vi "SVA_MAIN_2.vi"() -> ()   [LabVIEW 2021]
uses:
  Control-Case.ctl
  <vilib>/vision/NI_Vision_Development_Module.lvlib
panel:
  out "Distance 2":dbl[](graph) caption="Distancia entre perfil ideal y perfil real"
  out "Distance":dbl[](graph) caption="Distancia entre perfil ideal y perfil real"
  out "new picture 2":picture
  out "new picture":picture
  out "Datos finales":T1(array[cluster])
  in  "Crear patrón":bool
  in  "Concluir":bool
  in  "Lateral":bool
  in  "Superior":bool
  out "Fecha final":timestamp
  out "Rechazadas":dbl
  out "Aprobadas":dbl
  in  "Valor de aprobación Superiror":dbl=4.0 min=0.0 format="%.2f"
  out "Fecha inicio":timestamp
  out "Muestras":i16
  in  "Valor de aprobación Frontal":dbl=4.0 min=0.0 format="%.2f"
  # "Descripción:\nEste instrumento virtual permite detectar irregularidades en la geometría de latas de refresco usando el análisis de contornos:\n-Primeramente debe obtenerse un patrón para el perfil lateral e caso de no tenerlo, pues este se usará para detectar las irregularidades de capturas posteriores.\n-Como siguiente paso se toma una captura del perfil lateral y esta se desplegará en la imagen izquierda.\n-Como siguiente paso se toma una captura del perfil superior y esta se desplegará en la imagen derecha."
  # "Sistema de detección de defectos en latas \nbasado en el análisis de contornos\nProyecto de fin de semestre \nSistemas de visión artificial\nProfesor Erick Huitrón Ramírez"
  # "CUEVAS CERÓN SERGIO ALBERTO\nREYES PÉREZ JAVIER\nSALCEDO LICEA JUAN CARLOS"
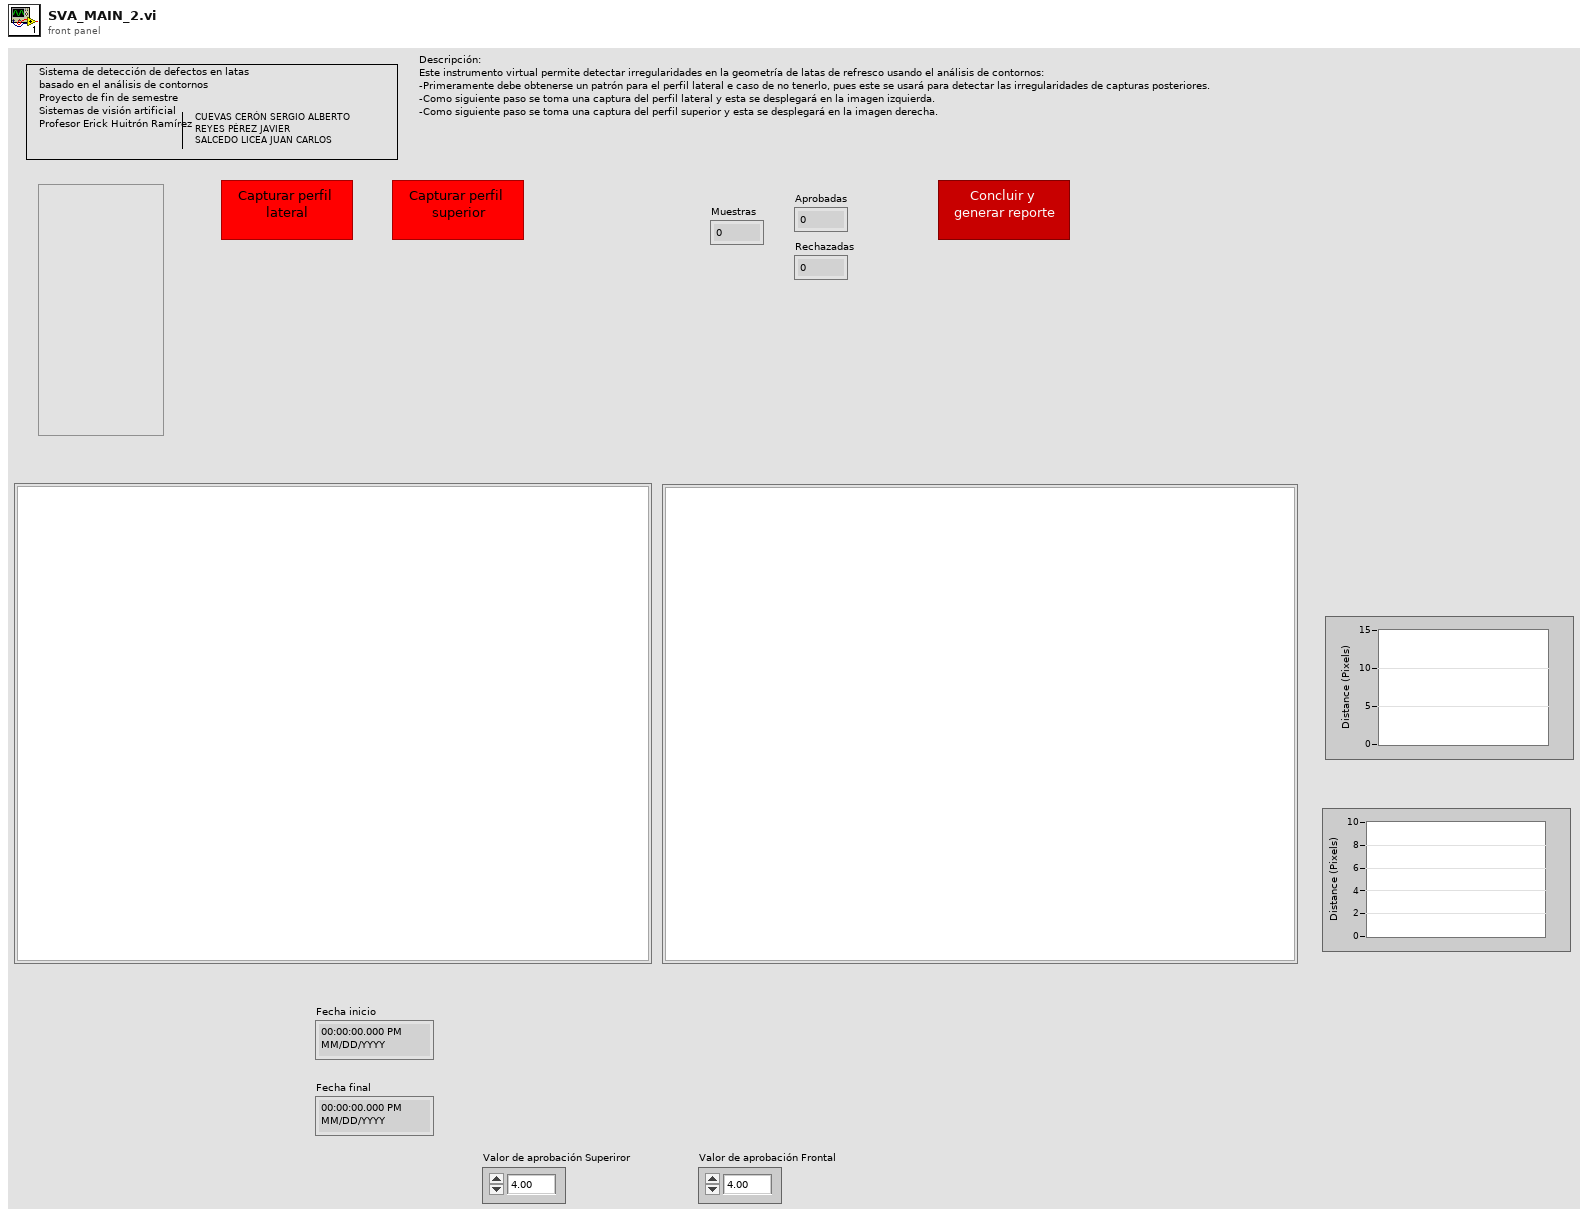
[diagram p1: front panel]
types:
  T1 = cluster{"Class":string, string, string, string}[]
  T2 = typedef "Control-Case.ctl" = enum16{"Espera", "Patrón", "Toma lateral", "Toma superior", "Concluir"}
  T3 = enum16{"Rect Left To Right", "Rect Right To Left", "Rect Top To Bottom", "Rect Bottom To Top", "Annulus Inner To Outer", "Annulus Outer To Inner", "Annulus Start Angle To End Angle", "Annulus End Angle To Start Angle"}
  T4 = enum16{"Closest To Search Start", "Maximum Length", "Strongest Mean Gradient Change"}
  T5 = cluster{"Overlay?":bool, "Color":u32, "Width":u32, "Maintain Width?":bool}
  T6 = typedef "IMAQ Rectangle" = cluster{"Left":i32, "Top":i32, "Right":i32, "Bottom":i32, "Rotation":dbl}
  T7 = typedef "IMAQ Image.ctl" = refnum<image>
  T8 = typedef "ROI Descriptor" = cluster{"Global Rectangle":i32[], "Contours":cluster{"ID":enum32{"External", "Internal"}, "Type":u32, "Coordinates":i32[]}[]}
  T9 = cluster{"Distance (Pixels)":dbl, "Distance (Real World)":dbl, "Angle (Absolute)":dbl, "Angle (Relative)":dbl}
  T10 = cluster{"Target Point":cluster{"X":dbl, "Y":dbl}, "Template Point":cluster{"X":dbl, "Y":dbl}, "Distance":dbl}[]
  T11 = cluster{"Class":string, "Distance (Pixels)":dbl, bool, "Distance (Pixels)":dbl}
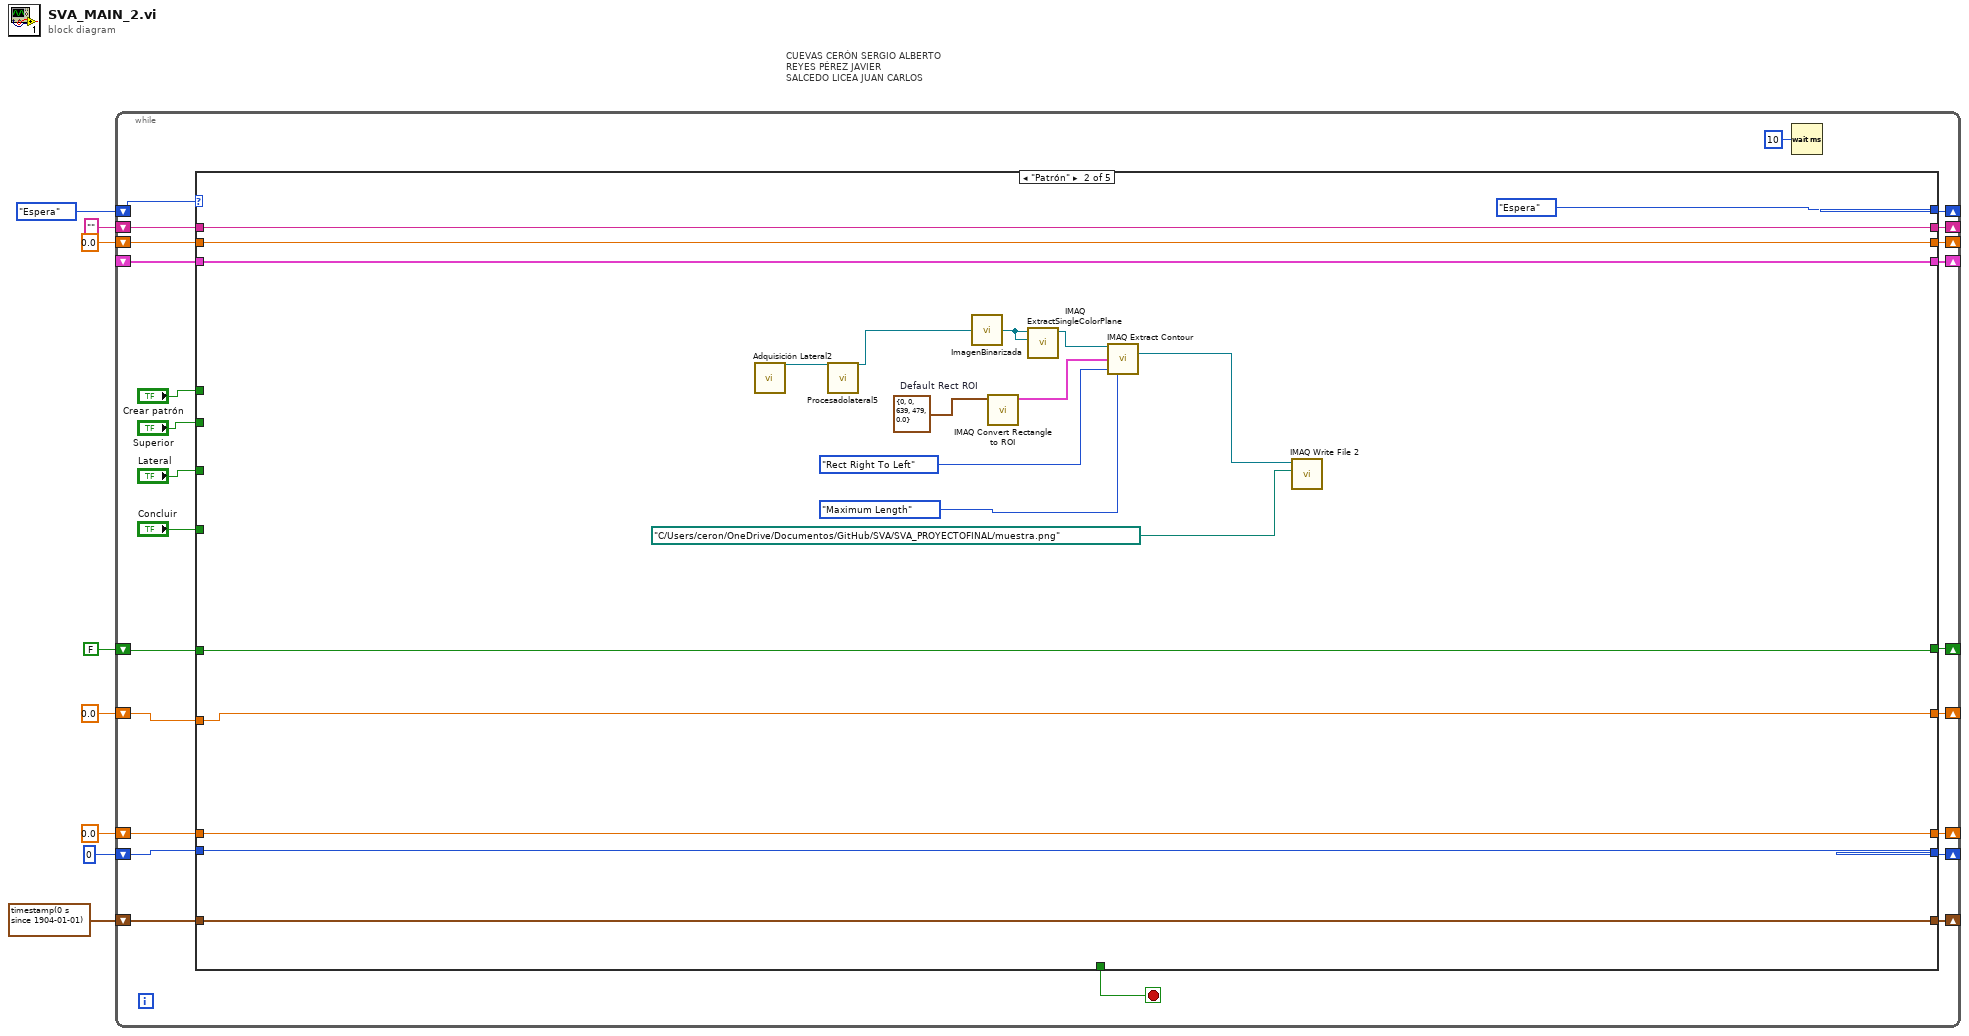
[diagram p0: block diagram]
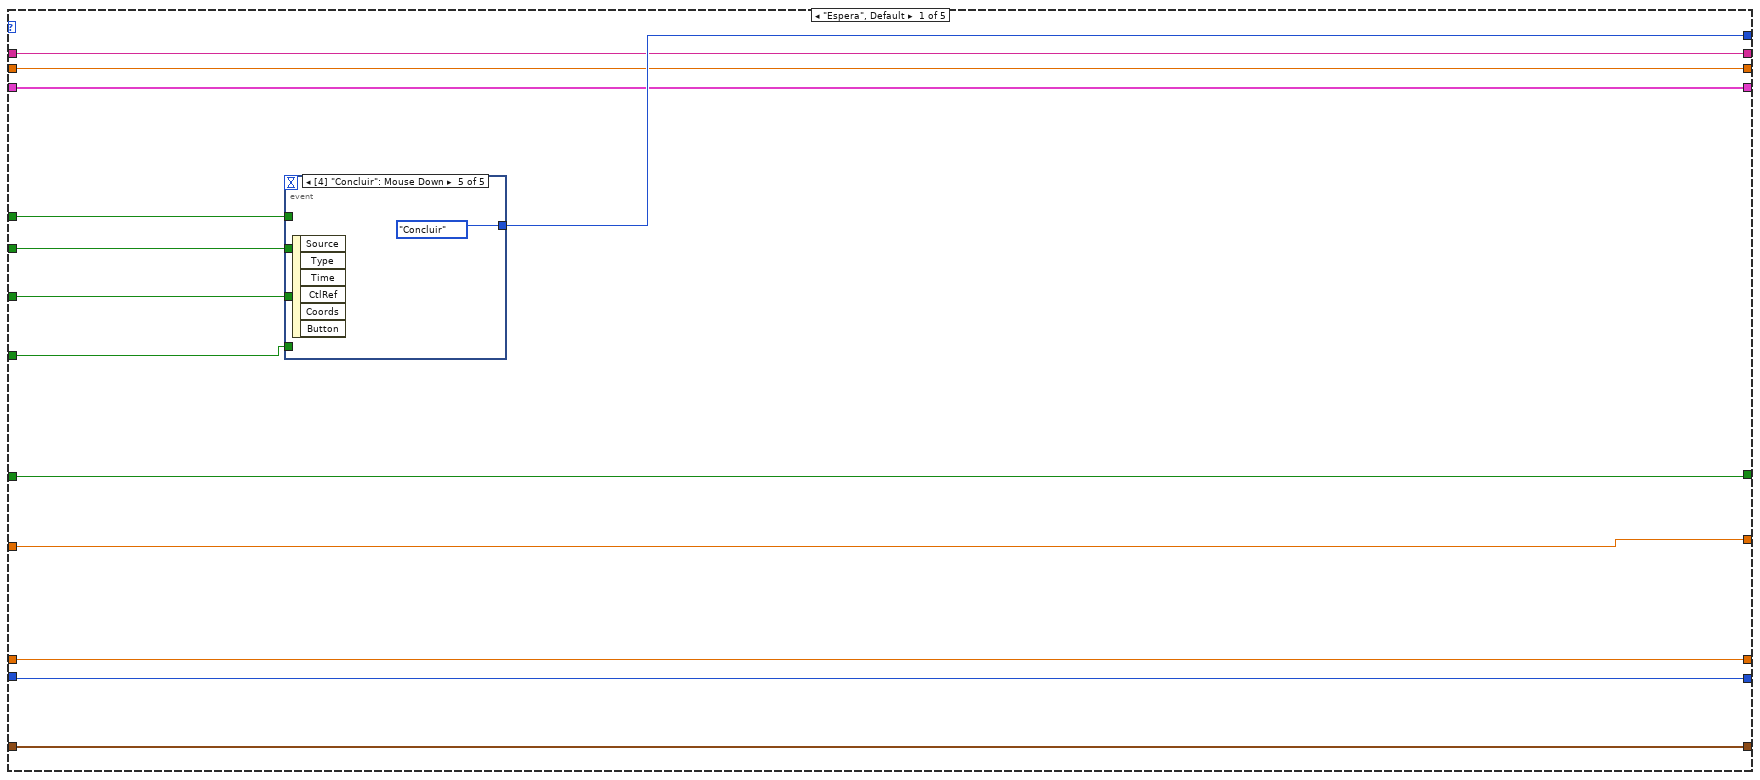
[diagram p2: hidden frame]
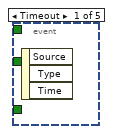
[diagram p3: hidden frame]
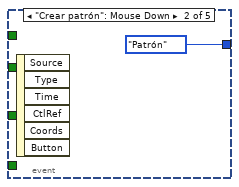
[diagram p4: hidden frame]
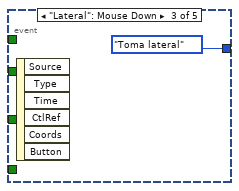
[diagram p5: hidden frame]
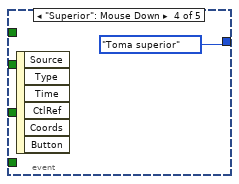
[diagram p6: hidden frame]
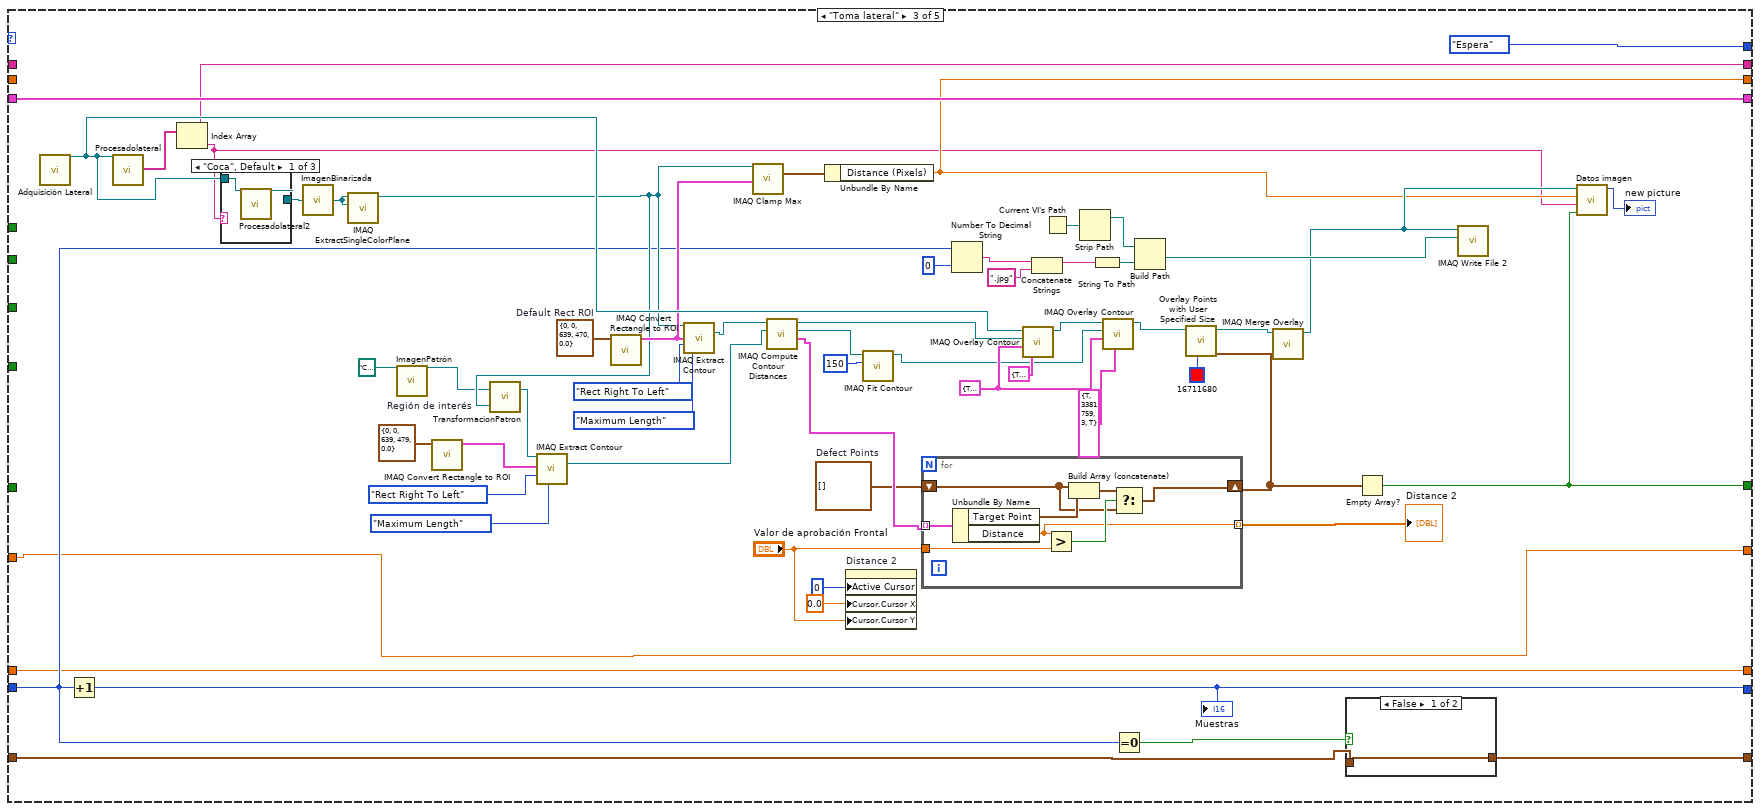
[diagram p7: hidden frame]
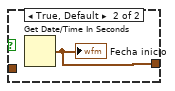
[diagram p8: hidden frame]
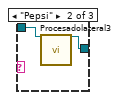
[diagram p9: hidden frame]
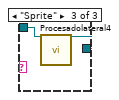
[diagram p10: hidden frame]
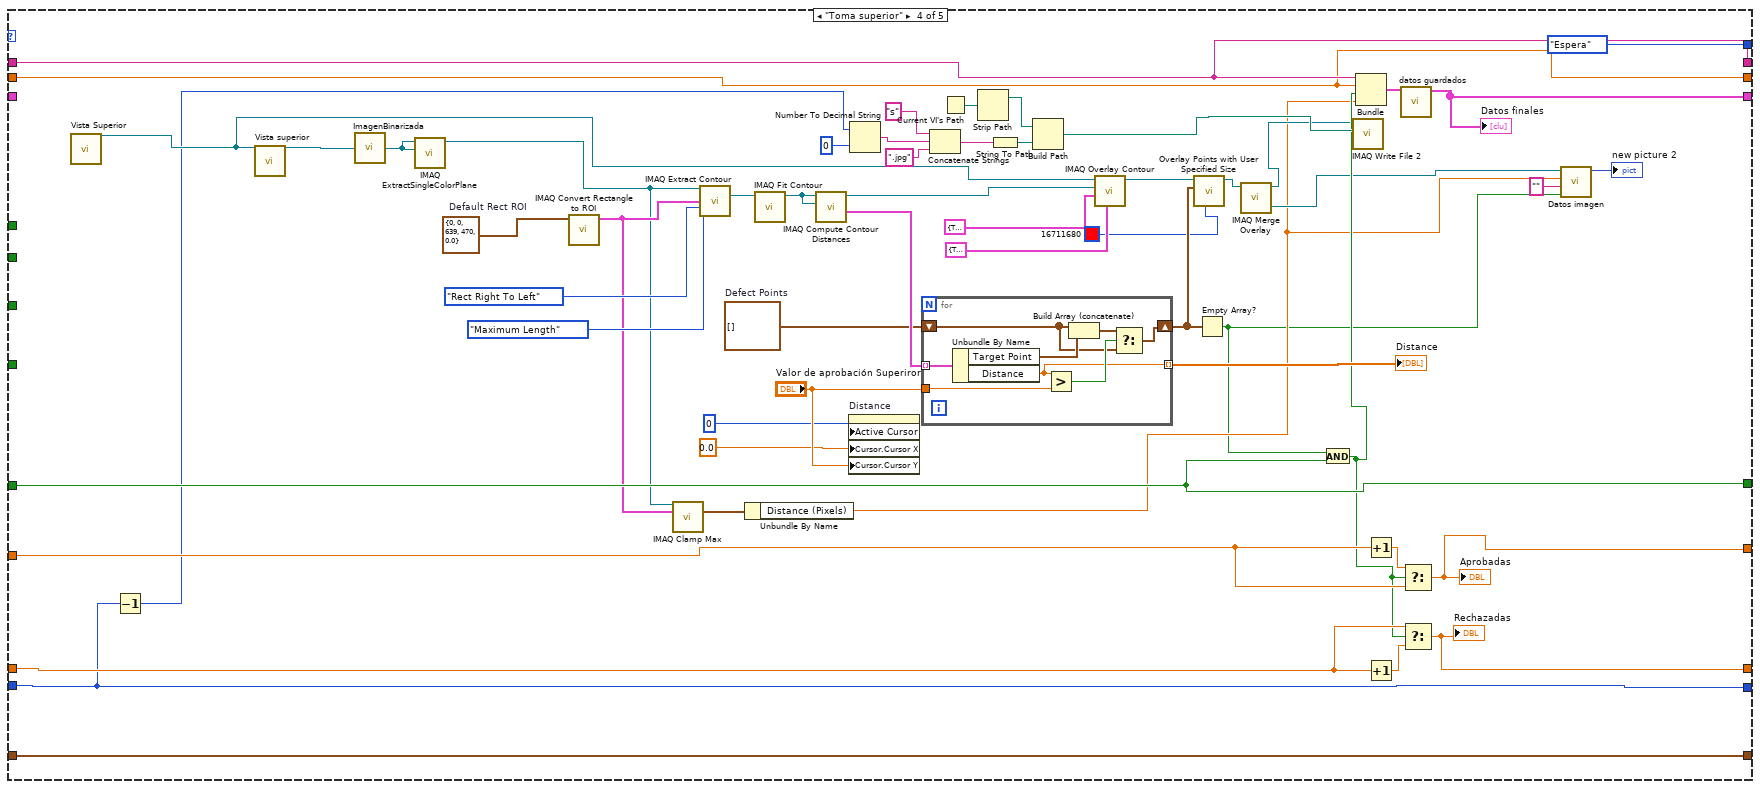
[diagram p11: hidden frame]
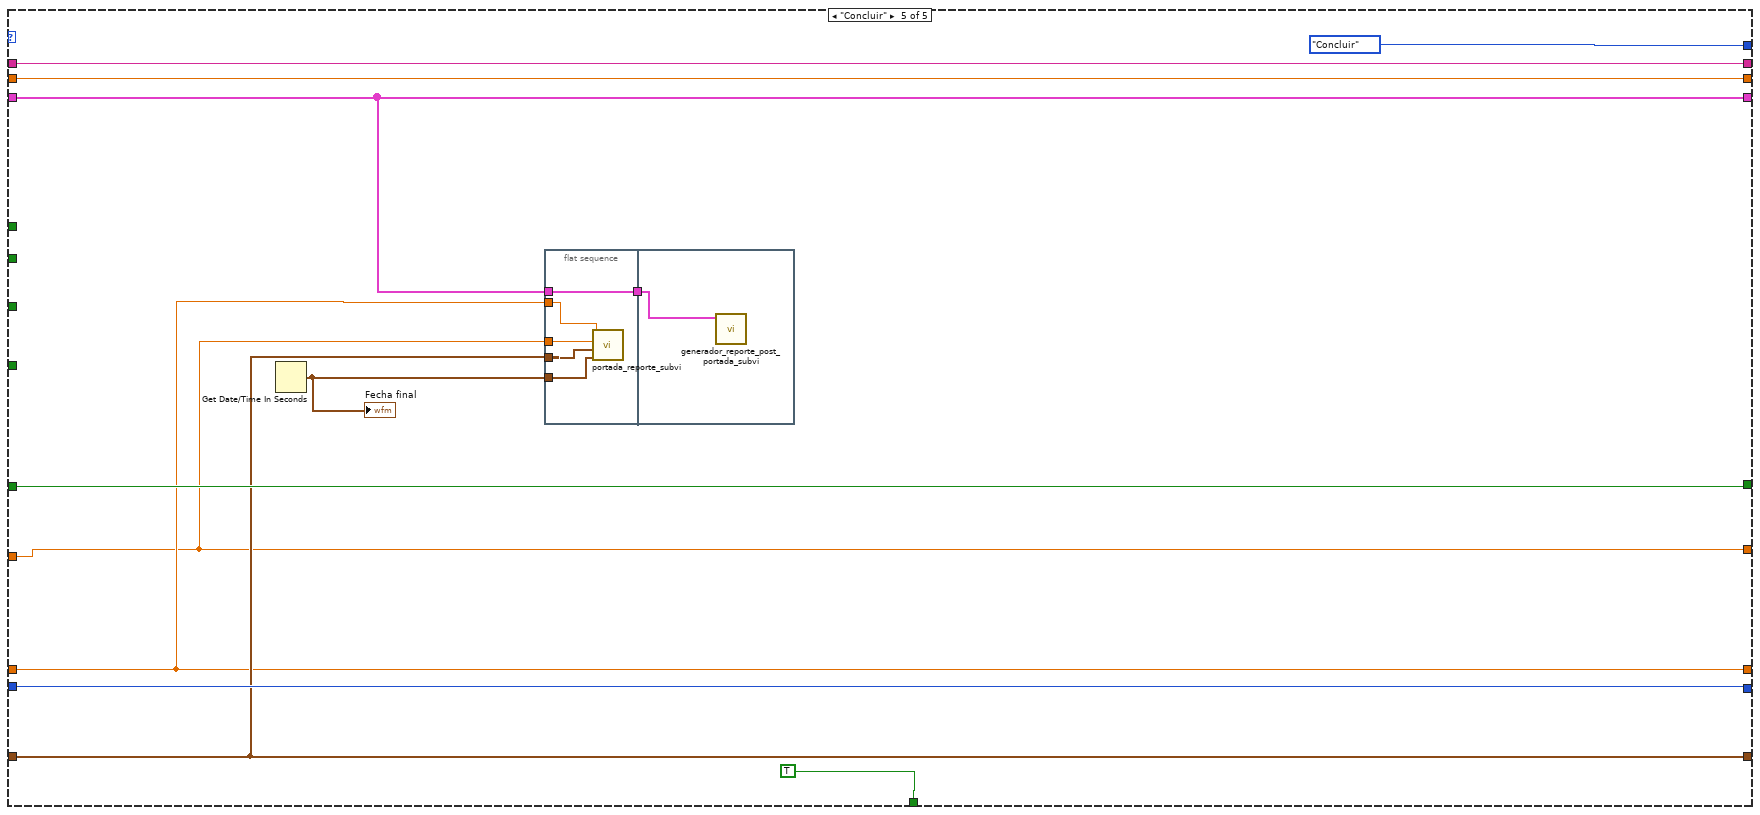
[diagram p12: hidden frame]
diagram:
  # "CUEVAS CERÓN SERGIO ALBERTO\nREYES PÉREZ JAVIER\nSALCEDO LICEA JUAN CARLOS"
  n1 = while {
    shift-right: [w32] -> _
    shift-left: Control-Case."Espera" -> [w31]
    shift-right: [w25] -> _
    shift-left: i16 0 ("x") -> [w24]
    shift-right: [w23] -> _
    shift-left: FALSE ("empty?") -> [w22]
    shift-right: [w21] -> _
    shift-left: 0.0 -> [w19]
    shift-right: [w20] -> _
    shift-left: 0.0 -> [w18]
    shift-right: [w16] -> _
    shift-left: 0.0 ("Distance (Pixels)") -> [w14]
    shift-right: [w17] -> _
    shift-left: "" ("Class") -> [w15]
    shift-right: [w13] -> _
    shift-left: _ -> [w12]
    shift-right: [w11] -> _
    shift-left: timestamp(0 s since 1904-01-01) ("seconds since 1Jan1904") -> [w10]
    stop <- w30 stop-if-true
    n2 = case shown="\"Patrón\"" w31 {
      tunnel: [w45 Control-Case."Espera" Control-Case."Espera" Control-Case."Espera" Control-Case."Concluir"] -> w32
      tunnel: [_ _ _ _ TRUE] -> w30
      tunnel: "Crear patrón" -> [w44 _ _ _ _]
      tunnel: "Concluir" -> [w43 _ _ _ _]
      tunnel: "Lateral" -> [w42 _ _ _ _]
      tunnel: "Superior" -> [w41 _ _ _ _]
      tunnel: w24 -> [w37 w54 w82 w157 w214]
      tunnel: [w37 w54 w83 w157 w214] -> w25
      tunnel: [w40 w57 w71 w172 w213] -> w23
      tunnel: w22 -> [w40 w57 _ w172 w213]
      tunnel: [w39 w56 w81 w167 w206] -> w21
      tunnel: [w38 w55 w80 w166 w207] -> w20
      tunnel: w19 -> [w39 w56 w81 w174 w206]
      tunnel: w18 -> [w38 w55 w80 w173 w207]
      tunnel: [w36 w53 w70 w171 w212] -> w17
      tunnel: [w35 w52 w72 w170 w211] -> w16
      tunnel: w15 -> [w36 w53 _ w171 w212]
      tunnel: w14 -> [w35 w52 _ w170 w211]
      tunnel: [w34 w51 w73 w169 w209] -> w13
      tunnel: w12 -> [w34 w51 w73 _ w209]
      tunnel: [w33 w50 w79 w168 w208] -> w11
      tunnel: w10 -> [w33 w50 w78 w168 w208]
      frame "Espera", Default {
        n3 = event shown="[4] \"Concluir\": Mouse Down" {
          selector: _ -> [_ _ _ _ _]
          dyn-events: _ -> [_ _ _ _ _]
          timeout: _ -> [_ _ _ _ _]
          tunnel: w44 -> [_ _ _ _ _]
          tunnel: w41 -> [_ _ _ _ _]
          tunnel: w42 -> [_ _ _ _ _]
          tunnel: w43 -> [_ _ _ _ _]
          tunnel: [_ Control-Case."Patrón" Control-Case."Toma lateral" Control-Case."Toma superior" Control-Case."Concluir"] -> w45
          event Timeout {
            n4 = event-data() -> ()  [unwired: 1 in, 3 out]
          }
          event "Crear patrón": Mouse Down {
            n5 = event-data() -> ()  [unwired: 1 in, 6 out]
          }
          event "Lateral": Mouse Down {
            n6 = event-data() -> ()  [unwired: 1 in, 6 out]
          }
          event "Superior": Mouse Down {
            n7 = event-data() -> ()  [unwired: 1 in, 6 out]
          }
          event "Concluir": Mouse Down {
            n8 = event-data() -> ()  [unwired: 1 in, 6 out]
          }
        }
      }
      frame "Patrón" {
        w65 = T6 {"Left"=0, "Top"=0, "Right"=639, "Bottom"=479, "Rotation"=0.0}  # Default Rect ROI
        n9 = call "Adquisición Lateral2"() -> ("Image Out"=w60:T7)  [unwired: 26 in, 1 out]
        n10 = call "Procesadolateral5"("Image In"=w60) -> ("Image Out"=w59:T7)  [unwired: 23 in, 3 out]
        n11 = call "ImagenBinarizada.vi"("Refnum in"=w59) -> ("Refnum out"=w61:T7)
        n12 = call "IMAQ Convert Rectangle to ROI"("Rectangle"=w65) -> ("ROI Descriptor"=w64:T8)  [unwired: 8 in, 1 out]
        n13 = call "IMAQ ExtractSingleColorPlane"("Image Dst"=w61, "Image Src"=w61) -> ("Image Dst Out"=w68:T7)  [unwired: 8 in, 1 out]
        n14 = call "IMAQ Extract Contour"("Source Image"=w68, "ROI Descriptor"=w64, "Search Direction"=T3."Rect Right To Left", "Contour Selection"=T4."Maximum Length") -> ("Contour Image Out"=w63:T7)  [unwired: 4 in, 7 out]
        n15 = call-poly "IMAQ Write File 2"("File Path"=path "C:/Users/ceron/OneDrive/Documentos/GitHub/SVA/SVA_PROYECTOFINAL/muestra.png" ("Imagen \nPatrón 2"), "Image"=w63) -> ()  [unwired: 8 in, 2 out]
      }
      frame "Toma lateral" {
        w87 = T6 {"Left"=0, "Top"=0, "Right"=639, "Bottom"=479, "Rotation"=0.0}  # Región de interés
        w89 = T6 {"Left"=0, "Top"=0, "Right"=639, "Bottom"=470, "Rotation"=0.0}  # Default Rect ROI
        w101 = cluster{"X":dbl, "Y":dbl}[] []  # Defect Points
        w97 = T5 {"Overlay?"=TRUE, "Color"=6618880, "Width"=3, "Maintain Width?"=TRUE} ("Contour Points Settings")
        n16 = call "Adquisición Lateral"() -> ("Image Out"=w127:T7)  [unwired: 26 in, 1 out]
        n17 = Increment(x=w82) -> (x+1=w83:i16)
        "Muestras" <- w83
        n18 = call "Procesadolateral"("Image In"=w127) -> ("Classes (TipoRefresco)"=w118:string[])  [unwired: 23 in, 3 out]
        n19 = Index Array(array=w118) -> (element=w70:string)  [unwired: 1 in]
        n20 = case shown="\"Coca\", Default" w70 {
          tunnel: w127 -> [w138 w141 w143]
          tunnel: [w139 w140 w142] -> w119
          frame "Coca", Default {
            n21 = call "Procesadolateral2"("Image In"=w138) -> ("Image Out"=w139:T7)  [unwired: 25 in, 1 out]
          }
          frame "Pepsi" {
            n22 = call "Procesadolateral3"("Image In"=w141) -> ("Image Out"=w140:T7)  [unwired: 25 in, 1 out]
          }
          frame "Sprite" {
            n23 = call "Procesadolateral4"("Image In"=w143) -> ("Image Out"=w142:T7)  [unwired: 25 in, 1 out]
          }
        }
        n24 = call "ImagenBinarizada.vi"("Refnum in"=w119) -> ("Refnum out"=w111:T7)
        n25 = call "IMAQ ExtractSingleColorPlane"("Image Dst"=w111, "Image Src"=w111) -> ("Image Dst Out"=w115:T7)  [unwired: 8 in, 1 out]
        n26 = call "ImagenPatrón"("Image Path"=path "C:/Users/ceron/OneDrive/Documentos/GitHub/SVA/SVA_PROYECTOFINAL/muestra.png" ("Imagen \nPatrón")) -> ("Image Out"=w110:T7)  [unwired: 25 in, 1 out]
        n27 = call "IMAQ Convert Rectangle to ROI"("Rectangle"=w87) -> ("ROI Descriptor"=w113:T8)  [unwired: 8 in, 1 out]
        n28 = call "TransformacionPatron.vi"("Patrón original"=w115, "Toma original"=w110) -> ("Toma corregida"=w114:T7)  [unwired: 1 out]
        n29 = call "IMAQ Extract Contour"("Source Image"=w114, "ROI Descriptor"=w113, "Search Direction"=T3."Rect Right To Left", "Contour Selection"=T4."Maximum Length") -> ("Contour Image Out"=w104:T7)  [unwired: 4 in, 7 out]
        n30 = call "IMAQ Convert Rectangle to ROI"("Rectangle"=w89) -> ("ROI Descriptor"=w116:T8)  [unwired: 8 in, 1 out]
        n31 = call "IMAQ Extract Contour"("Source Image"=w115, "ROI Descriptor"=w116, "Search Direction"=T3."Rect Right To Left", "Contour Selection"=T4."Maximum Length") -> ("Contour Image Out"=w103:T7)  [unwired: 4 in, 7 out]
        n32 = call "IMAQ Clamp Max"("Source Image"=w115, "ROI Descriptor"=w116) -> ("Clamp Results"=w117:T9)  [unwired: 8 in, 5 out]
        n33 = call "IMAQ Compute Contour Distances"("Template Contour Image"=w104, "Target Contour Image"=w103) -> ("Distances"=w106:T10, "Template Contour Image Out (dup)"=w107:T7, "Target Contour Image Out (dup)"=w109:T7)  [unwired: 3 in, 4 out]
        n34 = Unbundle By Name(w117) -> ("Distance (Pixels)"=w72:dbl)
        n35 = property on="Distance 2" class="WFGraph (strict)"("Active Cursor"=u32 0, "Cursor.Cursor X"=0.0 ("Cursor.Cursor Position:Cursor X"), "Cursor.Cursor Y"="Valor de aprobación Frontal") -> ()  [unwired: 2 in, 2 out]
        n36 = call-poly "IMAQ Fit Contour"("Control Points"=u32 150, "Contour Image"=w107) -> ("Contour Image Out"=w76:T7)  [unwired: 2 in, 7 out]
        n37 = for {
          tunnel: w106 -> [w130] mode=indexing
          shift-right: [w133] -> w112
          shift-left: w101 -> [w134]
          tunnel: [w132] -> w105 mode=indexing
          tunnel: "Valor de aprobación Frontal" -> [w131]
          n38 = Unbundle By Name(w130) -> ("Target Point"=w137:cluster{"X":dbl, "Y":dbl}, "Distance"=w132:dbl)
          n39 = Greater?(x=w132, y=w131) -> (0:w136:bool)
          n40 = Build Array (concatenate)(w134, w137) -> (w135:cluster{"X":dbl, "Y":dbl}[])
          n41 = Select(t=w135, s=w136, f=w134) -> (s? t:f=w133:cluster{"X":dbl, "Y":dbl}[])
        }
        "Distance 2" <- w105
        n42 = Number To Decimal String(number=w82, width (-)=i16 0) -> (decimal integer string=w123:string)
        n43 = call "IMAQ Overlay Contour"("Contour Equation Settings"=T5 {"Overlay?"=TRUE, "Color"=3381759, "Width"=3, "Maintain Width?"=TRUE}, "Contour Points Settings"=w97, "Contour Image"=w109, "Image"=w127) -> ("Image Out"=w108:T7)  [unwired: 2 in, 5 out]
        n44 = Concatenate Strings(w123, ".jpg" ("string")) -> (w124:string)
        n45 = Current VI's Path() -> (path=w122:path)
        n46 = Strip Path(path=w122) -> (stripped path=w121:path)  [unwired: 1 out]
        n47 = String To Path(string=w124) -> (path=w125:path)
        n48 = call "IMAQ Overlay Contour"("Contour Equation Settings"=T5 {"Overlay?"=TRUE, "Color"=3381759, "Width"=3, "Maintain Width?"=TRUE}, "Contour Points Settings"=w97, "Contour Image"=w76, "Image"=w108) -> ("Image Out"=w77:T7)  [unwired: 2 in, 5 out]
        n49 = Equal To 0?(x=w82) -> (x = 0?=w120:bool)
        n50 = Build Path(base path=w121, name or relative path=w125) -> (appended path=w126:path)
        n51 = call "Overlay Points with User Specified Size.vi"("Color"=u32 16711680, "Points"=w112, "Image In"=w77) -> ("Image Out"=w75:T7)  [unwired: 7 in, 1 out]
        n52 = call "IMAQ Merge Overlay"("Image Src"=w75) -> ("Image Dst Out"=w74:T7)  [unwired: 9 in, 1 out]
        n53 = case shown="False" w120 {
          tunnel: [w128 w129] -> w79
          tunnel: w78 -> [w128 _]
          frame False {
          }
          frame True, Default {
            n54 = Get Date/Time In Seconds() -> (seconds since 1Jan1904=w129:timestamp)
            "Fecha inicio" <- w129
          }
        }
        n55 = Empty Array?(array=w112) -> (empty?=w71:bool)
        n56 = call-poly "IMAQ Write File 2"("File Path"=w126, "Image"=w74) -> ()  [unwired: 8 in, 2 out]
        n57 = call "Datos imagen.vi"("Refnum in"=w74, "Distance (Pixels)"=w72, "Class"=w70, "empty?"=w71) -> ("new picture"=→"new picture":picture)  [unwired: 6 in]
      }
      frame "Toma superior" {
        w178 = T6 {"Left"=0, "Top"=0, "Right"=639, "Bottom"=470, "Rotation"=0.0}  # Default Rect ROI
        w186 = cluster{"X":dbl, "Y":dbl}[] []  # Defect Points
        n58 = call "Vista Superior"() -> ("Image Out"=w195:T7)  [unwired: 26 in, 1 out]
        n59 = Decrement(x=w157) -> (x-1=w156:i16)
        n60 = call "Vista superior"("Image In"=w195) -> ("Image Out"=w197:T7)  [unwired: 25 in, 1 out]
        n61 = call "ImagenBinarizada.vi"("Refnum in"=w197) -> ("Refnum out"=w196:T7)
        n62 = call "IMAQ ExtractSingleColorPlane"("Image Dst"=w196, "Image Src"=w196) -> ("Image Dst Out"=w144:T7)  [unwired: 8 in, 1 out]
        n63 = call "IMAQ Convert Rectangle to ROI"("Rectangle"=w178) -> ("ROI Descriptor"=w153:T8)  [unwired: 8 in, 1 out]
        n64 = call "IMAQ Clamp Max"("Source Image"=w144, "ROI Descriptor"=w153) -> ("Clamp Results"=w154:T9)  [unwired: 8 in, 5 out]
        n65 = call "IMAQ Extract Contour"("Source Image"=w144, "ROI Descriptor"=w153, "Search Direction"=T3."Rect Right To Left", "Contour Selection"=T4."Maximum Length") -> ("Contour Image Out"=w188:T7)  [unwired: 4 in, 7 out]
        n66 = Unbundle By Name(w154) -> ("Distance (Pixels)"=w148:dbl)
        n67 = call-poly "IMAQ Fit Contour"("Contour Image"=w188) -> ("Contour Image Out"=w194:T7)  [unwired: 3 in, 7 out]
        n68 = call "IMAQ Compute Contour Distances"("Template Contour Image"=w194, "Target Contour Image"=w194) -> ("Distances"=w193:T10, "Target Contour Image Out (dup)"=w187:T7)  [unwired: 3 in, 5 out]
        n69 = property on="Distance" class="WFGraph (strict)"("Active Cursor"=u32 0, "Cursor.Cursor X"=0.0 ("Cursor.Cursor Position:Cursor X"), "Cursor.Cursor Y"="Valor de aprobación Superiror") -> ()  [unwired: 2 in, 2 out]
        n70 = Number To Decimal String(number=w156, width (-)=i16 0) -> (decimal integer string=w163:string)
        n71 = for {
          tunnel: w193 -> [w205] mode=indexing
          shift-right: [w200] -> w190
          shift-left: w186 -> [w201]
          tunnel: [w199] -> w191 mode=indexing
          tunnel: "Valor de aprobación Superiror" -> [w198]
          n72 = Unbundle By Name(w205) -> ("Target Point"=w204:cluster{"X":dbl, "Y":dbl}, "Distance"=w199:dbl)
          n73 = Greater?(x=w199, y=w198) -> (0:w203:bool)
          n74 = Build Array (concatenate)(w201, w204) -> (w202:cluster{"X":dbl, "Y":dbl}[])
          n75 = Select(t=w202, s=w203, f=w201) -> (s? t:f=w200:cluster{"X":dbl, "Y":dbl}[])
        }
        "Distance" <- w191
        n76 = Concatenate Strings("s" ("string"), w163, ".jpg" ("string")) -> (w164:string)
        n77 = Current VI's Path() -> (path=w162:path)
        n78 = Strip Path(path=w162) -> (stripped path=w161:path)  [unwired: 1 out]
        n79 = String To Path(string=w164) -> (path=w165:path)
        n80 = Build Path(base path=w161, name or relative path=w165) -> (appended path=w155:path)
        n81 = call "IMAQ Overlay Contour"("Contour Equation Settings"=T5 {"Overlay?"=TRUE, "Color"=3381759, "Width"=3, "Maintain Width?"=TRUE}, "Contour Points Settings"=T5 {"Overlay?"=TRUE, "Color"=6618880, "Width"=3, "Maintain Width?"=TRUE}, "Contour Image"=w187, "Image"=w195) -> ("Image Out"=w192:T7)  [unwired: 2 in, 5 out]
        n82 = call "Overlay Points with User Specified Size.vi"("Color"=u32 16711680, "Points"=w190, "Image In"=w192) -> ("Image Out"=w151:T7)  [unwired: 7 in, 1 out]
        n83 = Empty Array?(array=w190) -> (empty?=w147:bool)
        n84 = call "IMAQ Merge Overlay"("Image Src"=w151) -> ("Image Dst Out"=w149:T7)  [unwired: 9 in, 1 out]
        n85 = And(x=w147, y=w172) -> (x .and. y?=w150:bool)
        n86 = call-poly "IMAQ Write File 2"("File Path"=w155, "Image"=w149) -> ()  [unwired: 8 in, 2 out]
        n87 = Bundle("Class"=w171, "Distance (Pixels)"=w170, w150, "Distance (Pixels)"=w148) -> (w152:T11)  [unwired: 1 in]
        n88 = Increment(x=w174) -> (x+1=w176:dbl)
        n89 = Increment(x=w173) -> (x+1=w175:dbl)
        n90 = call "datos guardados.vi"("Datos"=w152) -> ("appended array"=w169:T1)  [unwired: 10 in]
        "Datos finales" <- w169
        n91 = Select(t=w176, s=w150, f=w174) -> (s? t:f=w167:dbl)
        "Aprobadas" <- w167
        n92 = Select(t=w173, s=w150, f=w175) -> (s? t:f=w166:dbl)
        "Rechazadas" <- w166
        n93 = call "Datos imagen.vi"("Refnum in"=w149, "Distance (Pixels)"=w148, "Class"="", "empty?"=w147) -> ("new picture"=→"new picture 2":picture)  [unwired: 6 in]
      }
      frame "Concluir" {
        n94 = Get Date/Time In Seconds() -> (seconds since 1Jan1904=w217:timestamp)
        "Fecha final" <- w217
        n95 = flat-sequence {
          tunnel: w217 -> [w222]
          tunnel: w209 -> [w221]
          tunnel: [w221] -> w210
          tunnel: w208 -> [w220]
          tunnel: w207 -> [w219]
          tunnel: w206 -> [w218]
          tunnel: w210 -> [w223]
          frame #0 {
            n96 = call "portada_reporte_subvi.vi"("Final"=w222, "Inicio"=w220, "Numeric"=w218, "Numeric 2"=w219) -> ()  [unwired: 8 in]
          }
          frame #1 {
            n97 = call "generador_reporte_post_portada_subvi.vi"("Datos finales"=w223) -> ()  [unwired: 11 in]
          }
        }
      }
    }
    n98 = Wait (ms)(milliseconds to wait=u32 10) -> ()  [unwired: 1 out]
  }
